vi "Parse ERD Read Results (Rev 2 API).vi"(0 "Verify ERD Response?":bool=TRUE, 1 "Request ID":string, 2 "ERD Read Data In":T2 {"ERD Number" format="%.0x"}, 5 "Raw Message":string, 7 "Converted Data":T4 {"CRC" format="%04x"; "Length" format="%02x"; "Command" format="%02x"; "Destination" format="%02x"; "Source" format="%02x"}, 11 "Error In":errorcluster) -> (4 "Pass/Fail?":bool, 8 "ERD Read Data Out":T1 {"ERD Number" format="%.0x"}, 15 "Error Out":errorcluster)   [LabVIEW 2023, in "GEA2_Toolkit.lvlib"]
doc: "This VI takes the converted return data from the GEA2 Send and Receive and formats the Data based on the selections made in the Read ERD list. In addition, it also verifies the ERDs requested were returned."
uses:
  library/GEA2_Toolkit.lvlib
  type defs/Data Out.ctl
  type defs/ERD Read Data In.ctl
  type defs/Data Type.ctl
  type defs/ERD Read Data Out.ctl
panel:
  out "Command":u8 format="%x"
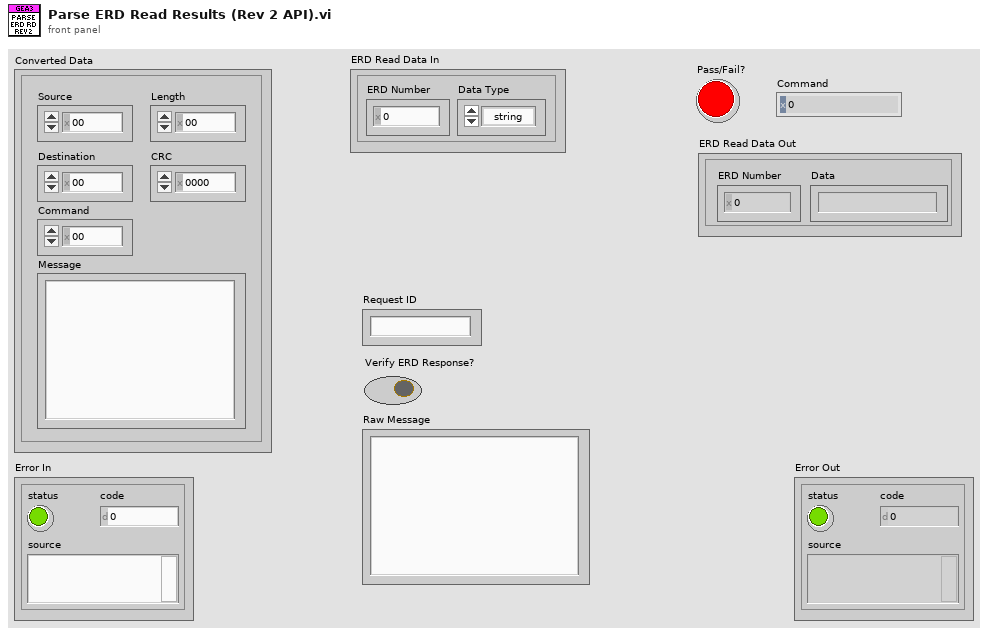
[diagram p1: front panel]
types:
  T1 = typedef "GEA2_Toolkit.lvlib/ERD Read Data Out.ctl" = cluster{"ERD Number":u16, "Data":string}
  T2 = typedef "GEA2_Toolkit.lvlib/ERD Read Data In.ctl" = cluster{"ERD Number":u16, "Data Type":T3}
  T3 = typedef "GEA2_Toolkit.lvlib/Data Type.ctl" = enum16{"string", "boolean", "uint8_t", "uint16_t", "uint32_t", "uint64_t", "int8_t", "int16_t", "int32_t", "int64_t"}
  T4 = typedef "GEA2_Toolkit.lvlib/Data Out.ctl" = cluster{"Source":u8, "Destination":u8, "Command":u8, "Length":u8, "CRC":u16, "Message":string}
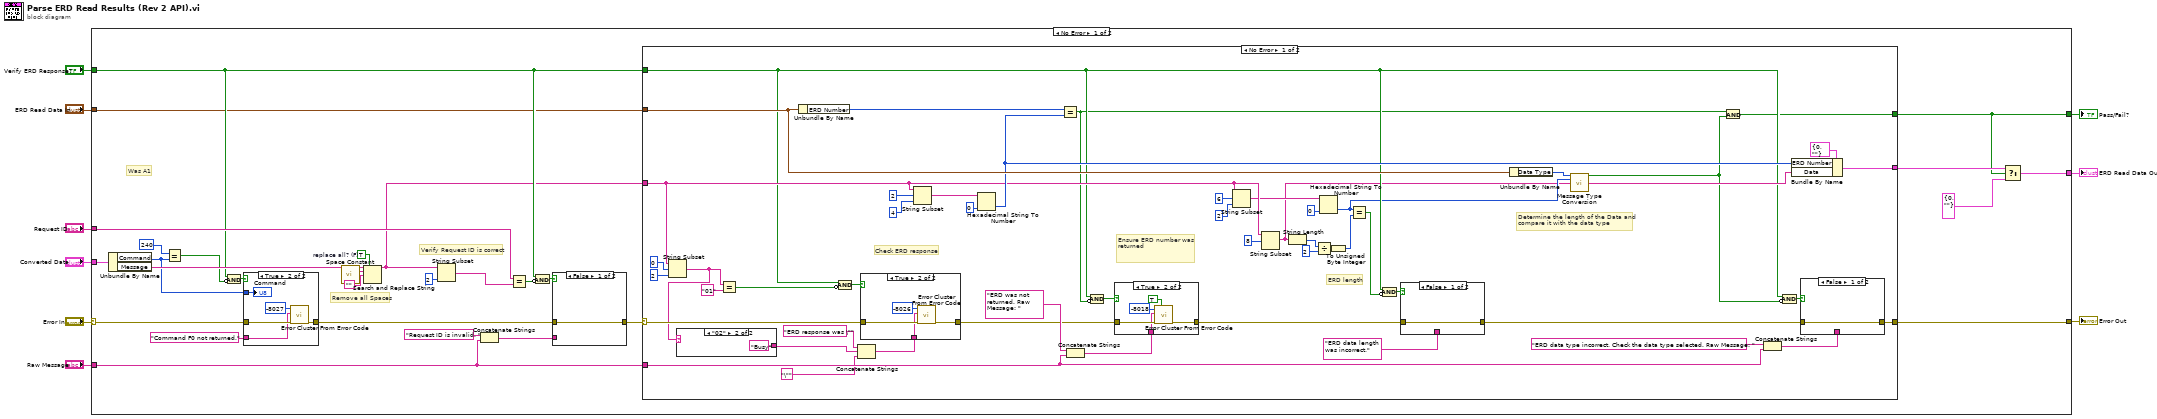
[diagram p0: block diagram]
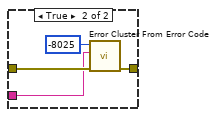
[diagram p3: hidden frame]
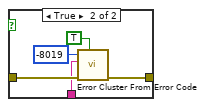
[diagram p4: hidden frame]
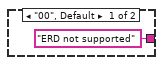
[diagram p5: hidden frame]
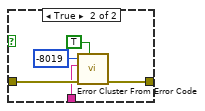
[diagram p8: hidden frame]
diagram:
  n1 = case shown="No Error" "Error In" {
    selector: "Error In" -> [w17 w128]
    tunnel: "Converted Data" -> [w38 _]
    tunnel: "ERD Read Data In" -> [w13 _]
    tunnel: [w21 _] -> w8
    tunnel: [w35 _] -> w1
    tunnel: [w30 w128] -> w6
    tunnel: "Raw Message" -> [w26 _]
    tunnel: "Verify ERD Response?" -> [w15 _]
    tunnel: "Request ID" -> [w23 _]
    frame No Error {
      w31 = TRUE  # replace all? (F)
      # "Was A1"
      # "Remove all Spaces"
      # "Verify Request ID is correct"
      n2 = Unbundle By Name(w38) -> ("Command"=w10:u8, "Message"=w32:string)
      n3 = Equal?(x=u8 240, y=w10) -> (x = y?=w16:bool)
      n4 = Compound Arithmetic op=AND(w15, invert w16) -> (w19:bool)
      n5 = case shown="True" w19 {
        tunnel: [w39 w44] -> w18
        tunnel: w17 -> [w39 w42]
        tunnel: "Command F0 not returned." -> [_ w41]
        tunnel: w10 -> [_ w40]
        frame False {
        }
        frame True {
          n6 = call <vilib>:"Error Cluster From Error Code.vi"("error in (no error)"=w42, "error message (\"\")"=w41, "error code (0)"=-8027) -> ("error out"=w44:errorcluster)  [unwired: 6 in]
          "Command" <- w40
        }
      }
      n7 = call <vilib>:"Space Constant.vi"() -> ("String"=w34:string)
      n8 = Search and Replace String(replace all?=w31, input string=w32, search string=w34, replace string="") -> (result string=w11:string)  [unwired: 4 in, 3 out]
      n9 = String Subset(string=w11, length (rest)=2 ("length (rest)")) -> (substring=w22:string)  [unwired: 1 in]
      n10 = Concatenate Strings("Request ID is invalid. " ("string"), w26) -> (w28:string)
      n11 = Equal?(x=w23, y=w22) -> (x = y?=w25:bool)
      n12 = Compound Arithmetic op=AND(w15, invert w25) -> (w24:bool)
      n13 = case shown="False" w24 {
        tunnel: [w45 w49] -> w27
        tunnel: w18 -> [w45 w47]
        tunnel: w28 -> [_ w46]
        frame False {
        }
        frame True {
          n14 = call <vilib>:"Error Cluster From Error Code.vi"("error in (no error)"=w47, "error message (\"\")"=w46, "error code (0)"=-8025) -> ("error out"=w49:errorcluster)  [unwired: 6 in]
        }
      }
      n15 = case shown="No Error" w27 {
        selector: w27 -> [w82 w127]
        tunnel: [w53 _] -> w21
        tunnel: w11 -> [w70 _]
        tunnel: w13 -> [w101 _]
        tunnel: [w52 _] -> w36
        tunnel: [w100 w127] -> w30
        tunnel: w26 -> [w99 _]
        tunnel: w15 -> [w60 _]
        frame No Error {
          # "ERD length"
          # "Check ERD response"
          # "Ensure ERD number was\nreturned"
          # "Determine the length of the Data and\ncompare it with the data type"
          n16 = String Subset(string=w70, offset (0)=0, length (rest)=2 ("length (rest)")) -> (substring=w79:string)
          n17 = case shown="\"02\"" w79 {
            tunnel: ["ERD not supported" ("string") "Busy" ("string")] -> w77
            frame "00", Default {
            }
            frame "02" {
            }
          }
          n18 = Equal?(x=w79, y="01") -> (x = y?=w81:bool)
          n19 = Unbundle By Name(w101) -> ("ERD Number"=w96:u16)
          n20 = Compound Arithmetic op=AND(w60, invert w81) -> (w80:bool)
          n21 = Concatenate Strings("ERD response was \"" ("string"), w77, "\"" ("string")) -> (w76:string)
          n22 = case shown="True" w80 {
            tunnel: [w110 w112] -> w83
            tunnel: w82 -> [w110 w113]
            tunnel: w76 -> [_ w111]
            frame False {
            }
            frame True {
              n23 = call <vilib>:"Error Cluster From Error Code.vi"("error in (no error)"=w113, "error message (\"\")"=w111, "error code (0)"=-8026) -> ("error out"=w112:errorcluster)  [unwired: 6 in]
            }
          }
          n24 = String Subset(string=w70, offset (0)=2, length (rest)=u32 4) -> (substring=w92:string)
          n25 = Hexadecimal String To Number(string=w92, default (0uL)=u16 0) -> (number=w95:u16)  [unwired: 1 in, 1 out]
          n26 = Equal?(x=w96, y=w95) -> (x = y?=w55:bool)
          n27 = Concatenate Strings("ERD was not returned. Raw Message: " ("string"), w99) -> (w89:string)
          n28 = Compound Arithmetic op=AND(w60, invert w55) -> (w87:bool)
          n29 = case shown="True" w87 {
            tunnel: [w115 w120] -> w63
            tunnel: w83 -> [w115 w119]
            tunnel: w89 -> [_ w116]
            frame False {
            }
            frame True {
              n30 = call <vilib>:"Error Cluster From Error Code.vi"("show call chain? (False)"=TRUE, "error in (no error)"=w119, "error message (\"\")"=w116, "error code (0)"=-8018) -> ("error out"=w120:errorcluster)  [unwired: 5 in]
            }
          }
          n31 = String Subset(string=w70, offset (0)=u32 6, length (rest)=2 ("length (rest)")) -> (substring=w69:string)
          n32 = String Subset(string=w70, offset (0)=u32 8) -> (substring=w56:string)  [unwired: 1 in]
          n33 = String Length(string=w56) -> (length=w67:i32)
          n34 = Divide(x=w67, y=2) -> (x/y=w65:dbl)
          n35 = Hexadecimal String To Number(string=w69, default (0uL)=u8 0 ("default (0 U32)")) -> (number=w57:u8)  [unwired: 1 in, 1 out]
          n36 = To Unsigned Byte Integer(number=w65) -> (unsigned 8bit integer=w64:u8)
          n37 = Equal?(x=w57, y=w64) -> (x = y?=w59:bool)
          n38 = Compound Arithmetic op=AND(w60, invert w59) -> (w61:bool)
          n39 = case shown="False" w61 {
            tunnel: [w102 w107] -> w62
            tunnel: w63 -> [w102 w106]
            tunnel: "ERD data length was incorrect." ("string") -> [_ w103]
            frame False {
            }
            frame True {
              n40 = call <vilib>:"Error Cluster From Error Code.vi"("show call chain? (False)"=TRUE, "error in (no error)"=w106, "error message (\"\")"=w103, "error code (0)"=-8019) -> ("error out"=w107:errorcluster)  [unwired: 5 in]
            }
          }
          n41 = Unbundle By Name(w101) -> ("Data Type"=w93:T3)
          n42 = call "Message Type Conversion.vi"("Data Type"=w93, "Data Length"=w57, "Message In"=w56) -> ("Pass/Fail?"=w54:bool, "Message Out"=w94:string)  [unwired: 11 in]
          n43 = Compound Arithmetic op=AND(w55, w54) -> (w53:bool)
          n44 = Concatenate Strings("ERD data type incorrect. Check the data type selected. Raw Message: " ("string"), w99) -> (w88:string)
          n45 = Compound Arithmetic op=AND(w60, invert w54) -> (w86:bool)
          n46 = Bundle By Name(cluster=T1 {"ERD Number"=0, "Data"=""} ("ERD Output"), "ERD Number"=w95, "Data"=w94) -> (w52:T1)
          n47 = case shown="False" w86 {
            tunnel: [w121 w126] -> w100
            tunnel: w62 -> [w121 w125]
            tunnel: w88 -> [_ w122]
            frame False {
            }
            frame True {
              n48 = call <vilib>:"Error Cluster From Error Code.vi"("show call chain? (False)"=TRUE, "error in (no error)"=w125, "error message (\"\")"=w122, "error code (0)"=-8019) -> ("error out"=w126:errorcluster)  [unwired: 5 in]
            }
          }
        }
        frame Error {
        }
      }
      n49 = Select(t=w36, s=w21, f=T1 {"ERD Number"=0, "Data"=""} ("ERD Output")) -> (s? t:f=w35:T1)
    }
    frame Error {
    }
  }
  "Pass/Fail?" <- w8
  "Error Out" <- w6
  "ERD Read Data Out" <- w1
